vi "Release Lock.vi"(7 "Lock Type":T1, 8 "error in (no error)":errorcluster, 11 "WebsocketStream in":refnum<class "WebsocketStream.lvclass">) -> (0 "error out":errorcluster, 3 "WebsocketStream out":refnum<class "WebsocketStream.lvclass">)   [LabVIEW 2020, in "Stream-Websocket.lvlib" / "WebsocketStream.lvclass"]
uses:
  WebsocketStream.lvclass
  Lock Type.ctl
  WebsocketStream.lvclass/WebsocketStream.ctl
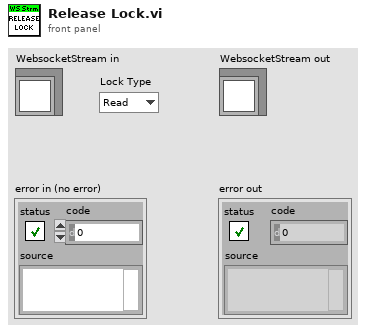
[diagram p1: front panel]
types:
  T1 = typedef "Stream-Websocket.lvlib/WebsocketStream.lvclass/Lock Type.ctl" = enum16{"Read", "Write"}
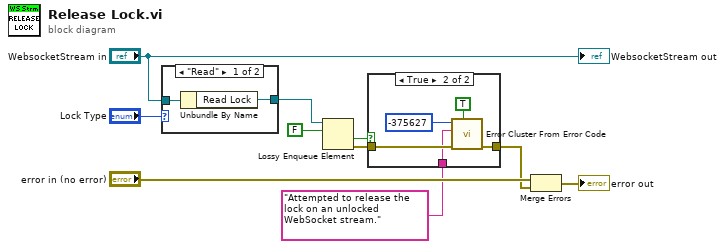
[diagram p0: block diagram]
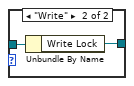
[diagram p2: hidden frame]
diagram:
  n1 = case shown="\"Read\"" "Lock Type" {
    tunnel: "WebsocketStream in" -> [w12 w14]
    tunnel: [w11 w13] -> w3
    frame "Read" {
      n2 = Unbundle By Name(w12) -> ("Read Lock"=w11:refnum<queue>)
    }
    frame "Write" {
      n3 = Unbundle By Name(w14) -> ("Write Lock"=w13:refnum<queue>)
    }
  }
  n4 = Lossy Enqueue Element(queue=w3, element=FALSE) -> (overflow?=w9:bool, error out=w8:errorcluster)  [unwired: 1 in, 2 out]
  n5 = case shown="True" w9 {
    tunnel: w8 -> [w15 w20]
    tunnel: [w15 w19] -> w6
    tunnel: "Attempted to release the lock on an unlocked WebSocket stream." -> [_ w16]
    frame False {
    }
    frame True {
      n6 = call <vilib>:"Error Cluster From Error Code.vi"("show call chain? (False)"=TRUE, "error in (no error)"=w20, "error message (\"\")"=w16, "error code (0)"=-375627) -> ("error out"=w19:errorcluster)  [unwired: 5 in]
    }
  }
  n7 = Merge Errors("error in (no error)", w6) -> (→"error out":errorcluster)
  "WebsocketStream out" <- "WebsocketStream in"
